vi "DI queue.vi"(5 "object":string="AZ1", 6 "DI state table":T1[](array[typedef]), 7 "date/time string":string, 8 "error in (no error)":errorcluster, 9 "discret parameters":bool[](array[boolean]), 10 "DI table":string[](array[string]), 11 "DI_msg":refnum<queue>) -> (0 "error out":errorcluster)   [LabVIEW 2019, in "Inputs.lvlib"]
uses:
  Inputs.lvlib
  Ctl/Parameter State.ctl
  Database/compress_discretes_1.vi/ee527a77-4d0f-4ded-954e-4d3d2a880cd4.vi
  Database/PostgreSQL.lvlib
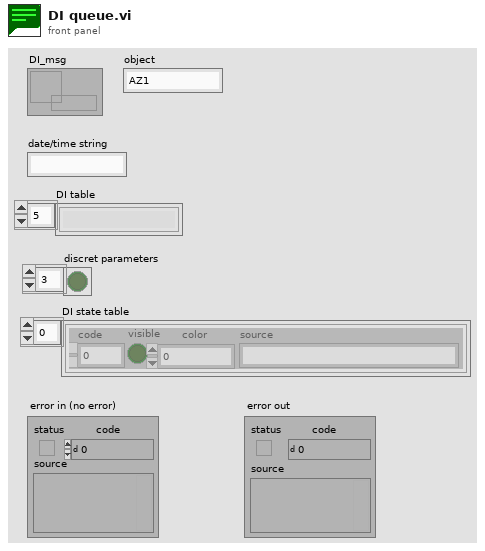
[diagram p1: front panel]
types:
  T1 = typedef "Inputs.lvlib/Parameter State.ctl" = cluster{"code":i32, "visible":bool, "color":u32, "source":string}
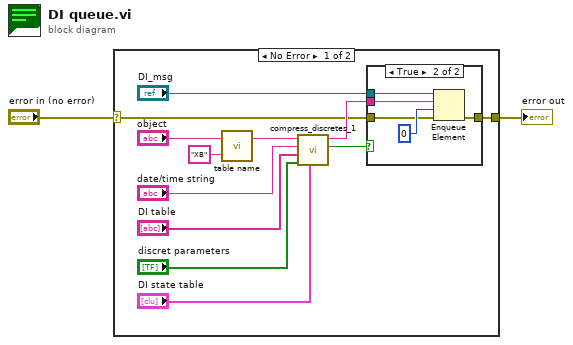
[diagram p0: block diagram]
diagram:
  n1 = case shown="No Error" "error in (no error)" {
    selector: "error in (no error)" -> [w4 w21]
    tunnel: [w10 w21] -> w1
    frame No Error {
      n2 = call "table name.vi"("postfix"="XB", "object name"="object") -> ("table name"=w7:string)  [unwired: 1 in]
      n3 = call "compress_discretes_1.vi"("DI state table"="DI state table", "discret parameters"="discret parameters", "DI table"="DI table", "date/time string"="date/time string", "table"=w7) -> ("Data to write"=w5:bool, "parameters"=w14:string)  [unwired: 5 in]
      n4 = case shown="True" w5 {
        tunnel: "DI_msg" -> [_ w19]
        tunnel: w14 -> [_ w18]
        tunnel: w4 -> [w15 w17]
        tunnel: [w15 w16] -> w10
        frame False {
        }
        frame True {
          n5 = Enqueue Element(queue=w19, element=w18, timeout in ms (-1)=0, error in (no error)=w17) -> (error out=w16:errorcluster)  [unwired: 2 out]
        }
      }
    }
    frame Error {
    }
  }
  "error out" <- w1
